vi "interfejsPC.vi"() -> ()   [LabVIEW 2014]
uses:
  glownaMaszynaStanowVIs/wczytajListePunktowVIs/RodzajPomiarow.ctl
  interfejsVIs/AkcjaInterfejsu.ctl
  glownaMaszynaStanowVIs/AkcjaGFV.ctl
  interfejsVIs/WejsciaVIs/WejsciaParametry.ctl
  interfejsVIs/WyjsciaVIs/WyjsciaParametry.ctl
panel:
  out "Połączono":bool
  in  "Połącz":bool
  in  "Port":u16=2000
  in  "Adres IP":string="192.168.0.102"
  in  "Wyjście":bool
  out "Odbiorcza azymut":i32
  out "Odbiorcza elewacja":i32
  out "Nadawcza azymut":i32
  out "Nadawcza elewacja":i32
  out "TCP Error":bool
  out "TCP Error Code":i32
  out "LINX Error Code":i32
  out "LINX Error":bool
  in  "Minimalna odległość":dbl=3.0
  in  "Długość ramienia":dbl=3.0
  in  "Testuj punkty":bool
  in  "Definicja punktów użytkownika:":i32[][](array[numeric])
  in  "Czas inicjalizacji ramion [s]":dbl=90.0
  in  "Czas pomiaru [s]":dbl=3.0
  in  "Rodzaj pomiarów:":T1
  out "Zrealizowano punkty:":string
  out "Pomiar":bool
  in  "Stop":bool
  in  "Start":bool
  out "Działanie ramienia":bool
  in  "Nadawcza/odbiorcza":bool
  out "Odb. góra":bool
  out "Odb. dół":bool
  out "Odb. prawo":bool
  out "Odb. lewo":bool
  in  "Dӣ":bool
  in  "GÓRA":bool
  in  "LEWO":bool
  in  "PRAWO":bool
  in  "Włącz/wyłącz":bool
  out "Nad. góra":bool
  out "Nad. dół":bool
  out "Nad. prawo":bool
  out "Nad. lewo":bool
  # "1. Podaj adres IP oraz port modułu sterującego. \nUstawione są domyślne wartości."
  # "Współrzędne kątowe ramion [st.]:"
  # "Informacje o błędach:"
  # "Ustawienia systemu.\nNajedź myszką na strzałki kontrolki aby\nprzeczytać opis."
  # "2. Wybierz rodzaj pomiarów:"
  # "3. Sprawdź ustawienia systemu i naciśnij \"Start\"."
  # "Komora nadawcza"
  # "Praca ręczna"
  # "Komora odbiorcza"
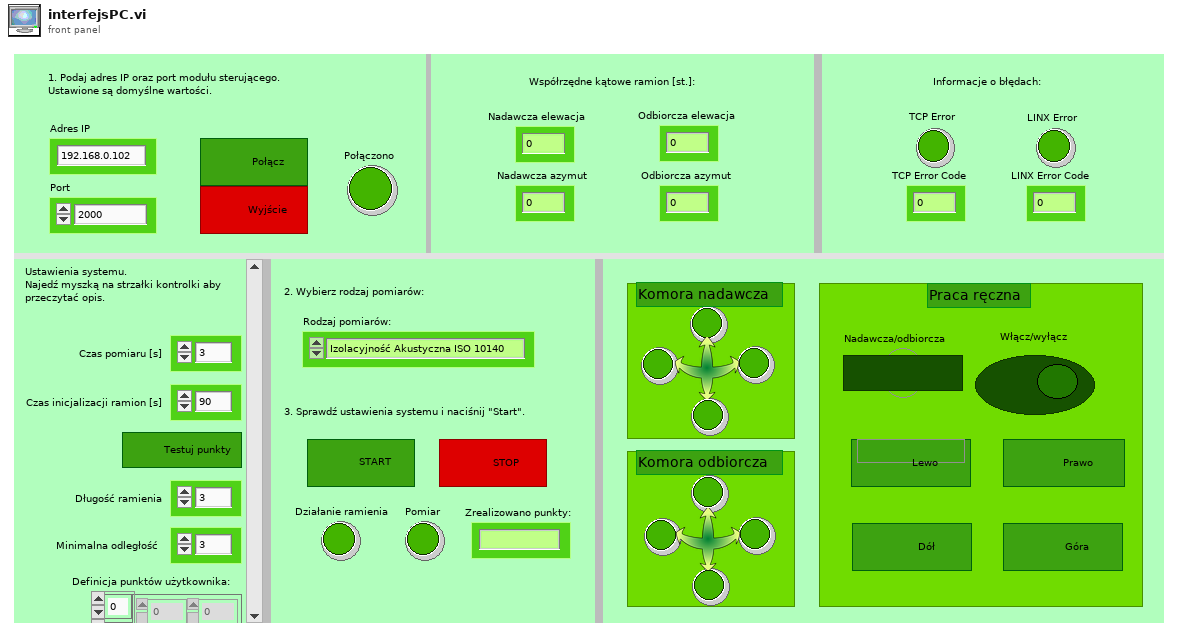
[diagram p1: front panel]
types:
  T1 = typedef "RodzajPomiarow.ctl" = enum16{"Izolacyjność Akustyczna ISO 10140", "Sekwencja testowa", "Definicja użytkownika"}
  T2 = typedef "AkcjaGFV.ctl" = enum16{"Czytaj", "Zapisz", "Reset"}
  T3 = typedef "AkcjaInterfejsu.ctl" = enum16{"Polacz", "Wczytaj", "Zapisz", "Koniec"}
  T4 = typedef "Odleglosc.ctl" = cluster{"Odległość [m]":dbl, "P1":i32[], "P2":i32[], "Czy poprawna":bool}
  T5 = typedef "WejsciaParametry.ctl" = cluster{"LEWO":bool, "PRAWO":bool, "GORA":bool, "DOL":bool, "Praca reczna":bool, "Stop":bool, "Start":bool, "Komora":bool, "Wyjscie":bool, "Rodzaj pomiarow":T1, "Czas pomiaru [s]":dbl, "Czas inicjalizacji ramion [s]":dbl, "Definicja punktów użytkownika":i32[][]}
  T6 = enum16{"Standard", "Buffered", "CRLF", "Immediate"}
  T7 = typedef "WyjsciaParametry.ctl" = cluster{"Nad. lewo":bool, "Nad.  prawo":bool, "Nad.  gora":bool, "Nad. doł":bool, "Dzialanie":bool, "Pomiar":bool, "Odb. lewo":bool, "Odb.  prawo":bool, "Odb.  gora":bool, "Odb. dol":bool, "Pozostalo punktow":i32, "Nad. elewacja":i32, "Nad. azymut":i32, "Odb. elewacja":i32, "Odb. azymut":i32, "TCP Error":bool, "TCP Error Code":i32, "LINX Error":bool, "LINX Error Code":i32}
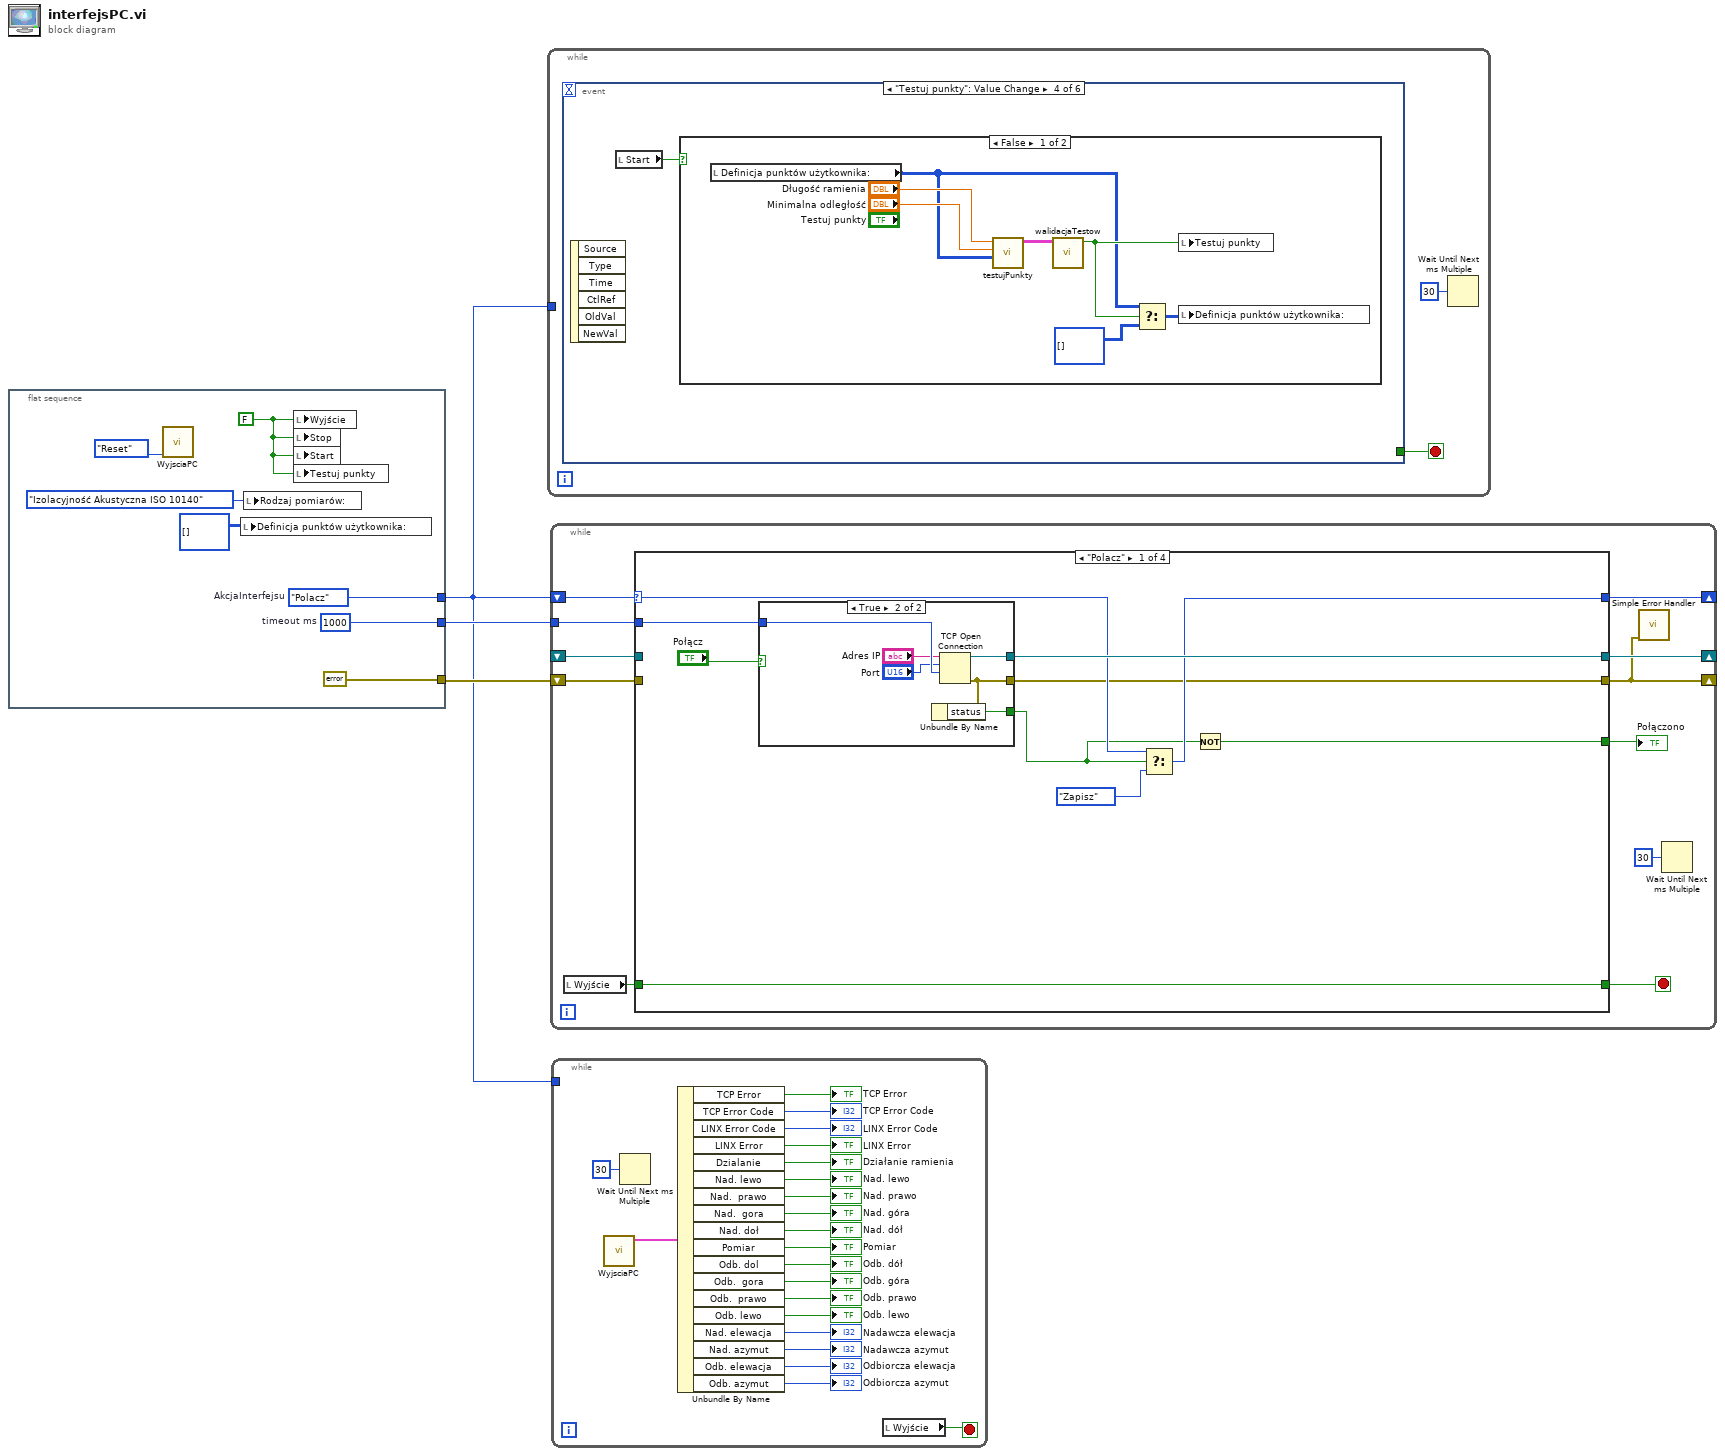
[diagram p0: block diagram]
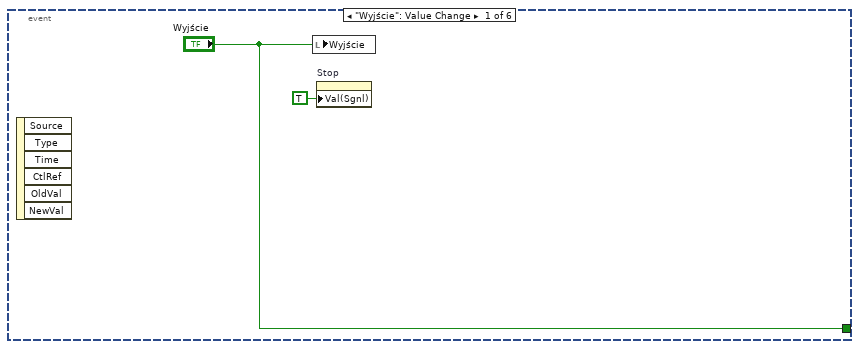
[diagram p2: hidden frame]
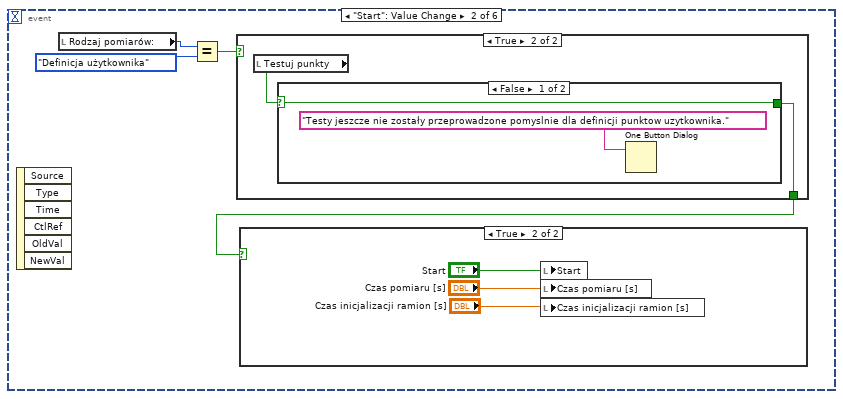
[diagram p3: hidden frame]
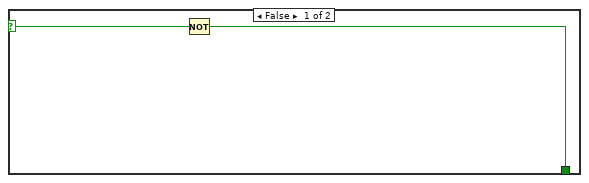
[diagram p5: hidden frame]
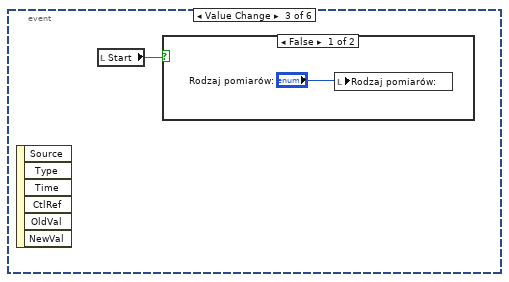
[diagram p7: hidden frame]
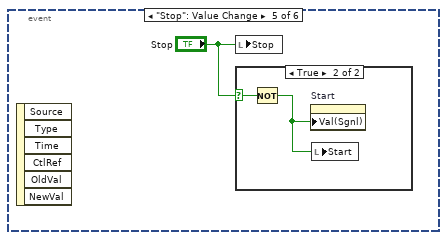
[diagram p10: hidden frame]
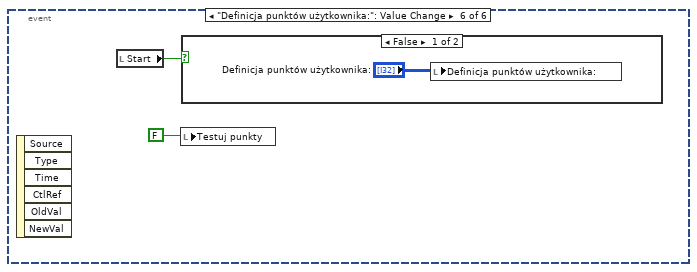
[diagram p12: hidden frame]
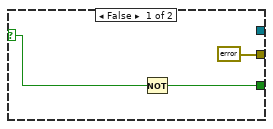
[diagram p14: hidden frame]
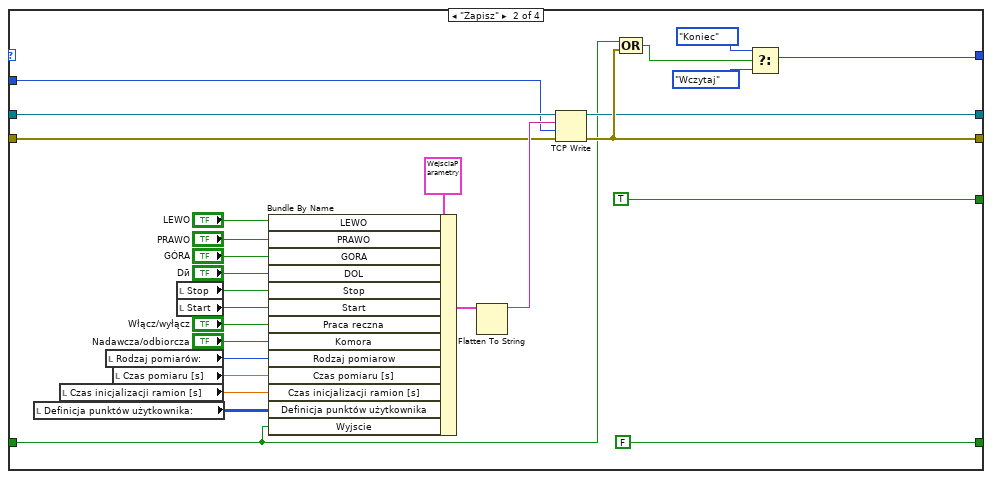
[diagram p15: hidden frame]
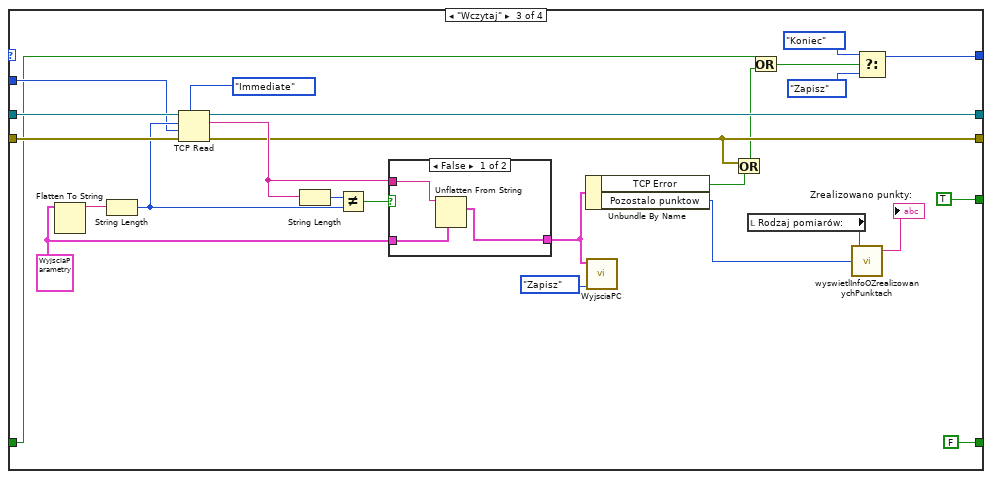
[diagram p16: hidden frame]
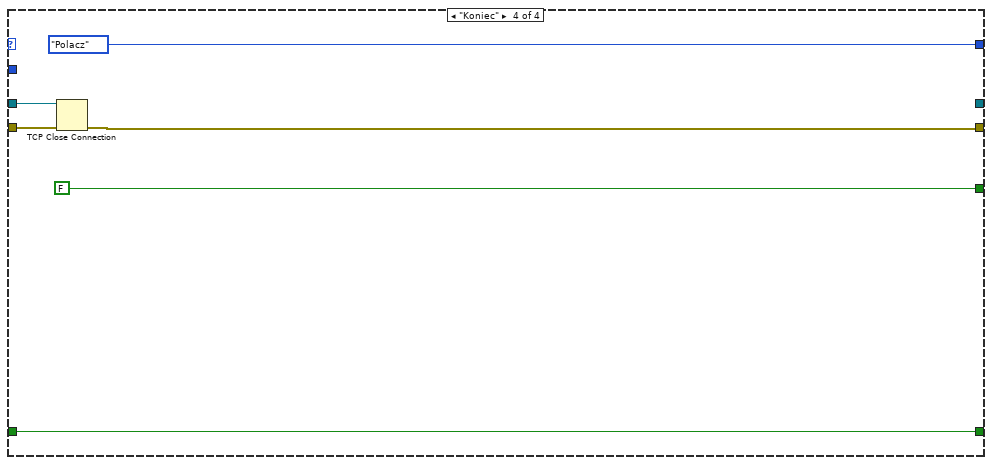
[diagram p18: hidden frame]
diagram:
  n1 = flat-sequence {
    tunnel: [w10] -> w1
    tunnel: [w9] -> w3
    tunnel: [errorcluster {"status"=FALSE, "code"=0, "source"=""} ("error out")] -> w2
    frame #0 {
      w5 = FALSE ("Wyjście")
      w9 = 1000  # timeout ms
      w10 = AkcjaInterfejsu."Polacz"  # AkcjaInterfejsu
      n2 = call "WyjsciaPC.vi"("Akcja"=AkcjaGFV."Reset") -> ()  [unwired: 10 in, 1 out]
      n3 = local write "Definicja punktów użytkownika:"(i32[][] [] ("Definicja punktów użytkownika")) -> ()
      n4 = local write "Rodzaj pomiarów:"(RodzajPomiarow."Izolacyjność Akustyczna ISO 10140" ("Rodzaj pomiarów:")) -> ()
      n5 = local write "Wyjście"(w5) -> ()
      n6 = local write "Stop"(w5) -> ()
      n7 = local write "Start"(w5) -> ()
      n8 = local write "Testuj punkty"(w5) -> ()
    }
  }
  n9 = while {
    tunnel: w1 -> [_]
    stop <- w12 stop-if-true
    n10 = event shown="[3] \"Testuj punkty\": Value Change" {
      selector: _ -> [_ _ _ _ _ _]
      dyn-events: _ -> [_ _ _ _ _ _]
      timeout: _ -> [_ _ _ _ _ _]
      tunnel: ["Wyjście" _ _ _ _ _] -> w12
      event "Wyjście": Value Change {
        n11 = event-data() -> ()  [unwired: 1 in, 6 out]
        n12 = local write "Wyjście"("Wyjście") -> ()
        n13 = property on="Stop" class="Bool (strict)"("Val(Sgnl)"=TRUE ("Value (Signaling)")) -> ()  [unwired: 2 in, 2 out]
      }
      event "Start": Value Change {
        n14 = event-data() -> ()  [unwired: 1 in, 6 out]
        n15 = local read "Rodzaj pomiarów:"() -> (w18:T1)
        n16 = Equal?(x=w18, y=RodzajPomiarow."Definicja użytkownika") -> (x = y?=w16:bool)
        n17 = case shown="True" w16 {
          selector: w16 -> [w23 _]
          tunnel: [w22 w24] -> w15
          frame False {
            n18 = Not(x=w23) -> (.not. x?=w22:bool)
          }
          frame True {
            n19 = local read "Testuj punkty"() -> (w25:bool)
            n20 = case shown="False" w25 {
              selector: w25 -> [w26 w28]
              tunnel: [w26 w28] -> w24
              frame False {
                n21 = One Button Dialog(message="Testy jeszcze nie zostały przeprowadzone pomyslnie dla definicji punktow uzytkownika.") -> ()  [unwired: 1 in, 1 out]
              }
              frame True {
              }
            }
          }
        }
        n22 = case shown="True" w15 {
          frame False {
          }
          frame True {
            n23 = local write "Start"("Start") -> ()
            n24 = local write "Czas pomiaru [s]"("Czas pomiaru [s]") -> ()
            n25 = local write "Czas inicjalizacji ramion [s]"("Czas inicjalizacji ramion [s]") -> ()
          }
        }
      }
      event Value Change {
        n26 = event-data() -> ()  [unwired: 1 in, 6 out]
        n27 = local read "Start"() -> (w29:bool)
        n28 = case shown="False" w29 {
          frame False {
            n29 = local write "Rodzaj pomiarów:"("Rodzaj pomiarów:") -> ()
          }
          frame True {
          }
        }
      }
      event "Testuj punkty": Value Change {
        n30 = event-data() -> ()  [unwired: 1 in, 6 out]
        n31 = local read "Start"() -> (w31:bool)
        n32 = case shown="False" w31 {
          frame False {
            n33 = local read "Definicja punktów użytkownika:"() -> (w32:i32[][])
            n34 = call "testujPunkty.vi"("Punkty"=w32, "Minimalna odległość"="Minimalna odległość", "Promień [m]"="Długość ramienia") -> ("Odleglosci"=w36:T4[][])  [unwired: 8 in]
            n35 = call "walidacjaTestow.vi"("Odleglosci"=w36) -> ("Testy przeszły?"=w35:bool)  [unwired: 10 in]
            n36 = Select(t=w32, s=w35, f=i32[][] []) -> (s? t:f=w33:i32[][])
            n37 = local write "Testuj punkty"(w35) -> ()
            n38 = local write "Definicja punktów użytkownika:"(w33) -> ()
          }
          frame True {
          }
        }
      }
      event "Stop": Value Change {
        n39 = event-data() -> ()  [unwired: 1 in, 6 out]
        n40 = local write "Stop"("Stop") -> ()
        n41 = case shown="True" "Stop" {
          selector: "Stop" -> [_ w41]
          frame False {
          }
          frame True {
            n42 = Not(x=w41) -> (.not. x?=w40:bool)
            n43 = property on="Start" class="Bool (strict)"("Val(Sgnl)"=w40) -> ()  [unwired: 2 in, 2 out]
            n44 = local write "Start"(w40) -> ()
          }
        }
      }
      event "Definicja punktów użytkownika:": Value Change {
        n45 = event-data() -> ()  [unwired: 1 in, 6 out]
        n46 = local read "Start"() -> (w42:bool)
        n47 = local write "Testuj punkty"(FALSE ("Testuj punkty")) -> ()
        n48 = case shown="False" w42 {
          frame False {
            n49 = local write "Definicja punktów użytkownika:"("Definicja punktów użytkownika:") -> ()
          }
          frame True {
          }
        }
      }
    }
    n50 = Wait Until Next ms Multiple(millisecond multiple=u32 30) -> ()  [unwired: 1 out]
  }
  n51 = while {
    shift-right: [w54] -> _
    shift-left: _ -> [w55]
    shift-right: [w46] -> _
    shift-left: w2 -> [w53]
    shift-right: [w49] -> _
    shift-left: w1 -> [w51]
    tunnel: w3 -> [w50]
    stop <- w52 stop-if-true
    n52 = local read "Wyjście"() -> (w48:bool)
    n53 = case shown="\"Polacz\"" w51 {
      selector: w51 -> [w60 _ _ _]
      tunnel: w55 -> [_ w101 w123 w137]
      tunnel: [w65 w85 w120 _] -> w54
      tunnel: [w57 w86 w109 w132] -> w46
      tunnel: w53 -> [_ w91 w124 w136]
      tunnel: [w63 FALSE ("Dzialanie") FALSE ("Wyjście") w134] -> w52
      tunnel: [w61 w90 w113 AkcjaInterfejsu."Polacz" ("AkcjaInterfejsu")] -> w49
      tunnel: w48 -> [w63 w75 w108 w134]
      tunnel: w50 -> [w62 w87 w121 _]
      tunnel: [w58 TRUE ("Wyjście") TRUE ("Wyjście") FALSE ("Wyjście")] -> w47
      frame "Polacz" {
        n54 = case shown="True" "Połącz" {
          selector: "Połącz" -> [w68 _]
          tunnel: [_ w74] -> w65
          tunnel: [errorcluster {"status"=FALSE, "code"=0, "source"=""} ("error out") w69] -> w57
          tunnel: w62 -> [_ w73]
          tunnel: [w66 w70] -> w56
          frame False {
            n55 = Not(x=w68) -> (.not. x?=w66:bool)
          }
          frame True {
            n56 = TCP Open Connection(address="Adres IP", remote port or service name="Port", timeout ms (60000)=w73) -> (connection ID=w74:refnum<k5>, error out=w69:errorcluster)  [unwired: 2 in]
            n57 = Unbundle By Name(w69) -> ("status"=w70:bool)
          }
        }
        n58 = Select(t=w60, s=w56, f=AkcjaInterfejsu."Zapisz" ("AkcjaInterfejsu")) -> (s? t:f=w61:T3)
        n59 = Not(x=w56) -> (.not. x?=w58:bool)
      }
      frame "Zapisz" {
        n60 = local read "Definicja punktów użytkownika:"() -> (w76:i32[][])
        n61 = local read "Czas inicjalizacji ramion [s]"() -> (w77:dbl)
        n62 = local read "Rodzaj pomiarów:"() -> (w82:T1)
        n63 = local read "Czas pomiaru [s]"() -> (w78:dbl)
        n64 = local read "Stop"() -> (w81:bool)
        n65 = local read "Start"() -> (w83:bool)
        n66 = Bundle By Name(cluster=T5 {"LEWO"=FALSE, "PRAWO"=FALSE, "GORA"=FALSE, "DOL"=FALSE, "Praca reczna"=FALSE, "Stop"=FALSE, "Start"=FALSE, "Komora"=FALSE, "Wyjscie"=FALSE, "Rodzaj pomiarow"=enum."Izolacyjność Akustyczna ISO 10140", "Czas pomiaru [s]"=2.0, "Czas inicjalizacji ramion [s]"=2.0, "Definicja punktów użytkownika"=[]} ("Wejścia interfejsu"), "LEWO"="LEWO", "PRAWO"="PRAWO", "GORA"="GÓRA", "DOL"="Dӣ", "Stop"=w81, "Start"=w83, "Praca reczna"="Włącz/wyłącz", "Komora"="Nadawcza/odbiorcza", "Rodzaj pomiarow"=w82, "Czas pomiaru [s]"=w78, "Czas inicjalizacji ramion [s]"=w77, "Definicja punktów użytkownika"=w76, "Wyjscie"=w75) -> (w93:T5)
        n67 = Flatten To String(anything=w93) -> (data string=w92:string)  [unwired: 3 in, 2 out]
        n68 = TCP Write(connection ID=w101, data in=w92, error in (no error)=w91, 9:w87) -> (connection ID out=w85:refnum<k5>, error out=w86:errorcluster)  [unwired: 1 out]
        n69 = Compound Arithmetic op=OR(w75, w86) -> (w88:bool)
        n70 = Select(t=AkcjaInterfejsu."Koniec", s=w88, f=AkcjaInterfejsu."Wczytaj") -> (s? t:f=w90:T3)
      }
      frame "Wczytaj" {
        w116 = T7 {"Nad. lewo"=FALSE, "Nad.  prawo"=FALSE, "Nad.  gora"=FALSE, "Nad. doł"=FALSE, "Dzialanie"=FALSE, "Pomiar"=FALSE, "Odb. lewo"=FALSE, "Odb.  prawo"=FALSE, "Odb.  gora"=FALSE, "Odb. dol"=FALSE, "Pozostalo punktow"=0, "Nad. elewacja"=0, "Nad. azymut"=0, "Odb. elewacja"=0, "Odb. azymut"=0, "TCP Error"=FALSE, "TCP Error Code"=0, "LINX Error"=FALSE, "LINX Error Code"=0} ("Cluster")
        n71 = Flatten To String(anything=w116) -> (data string=w126:string)  [unwired: 3 in, 2 out]
        n72 = String Length(string=w126) -> (length=w122:i32)
        n73 = TCP Read(connection ID=w123, bytes to read=w122, error in (no error)=w124, 7:T6."Immediate" ("mode (standard)"), 9:w121) -> (connection ID out=w120:refnum<k5>, data out=w117:string, error out=w109:errorcluster)
        n74 = String Length(string=w117) -> (length=w125:i32)
        n75 = Not Equal?(x=w125, y=w122) -> (x != y?=w118:bool)
        n76 = case shown="False" w118 {
          tunnel: w117 -> [w129 _]
          tunnel: w116 -> [w130 w131]
          tunnel: [w128 w131] -> w104
          frame False {
            n77 = Unflatten From String(type=w130, binary string=w129) -> (value=w128:T7)  [unwired: 3 in, 2 out]
          }
          frame True {
          }
        }
        n78 = Unbundle By Name(w104) -> ("TCP Error"=w103:bool, "Pozostalo punktow"=w102:i32)
        n79 = call "WyjsciaPC.vi"("Akcja"=AkcjaGFV."Zapisz", "Wejście"=w104) -> ()  [unwired: 9 in, 1 out]
        n80 = Or(x=w109, y=w103) -> (x .or. y?=w106:bool)
        n81 = local read "Rodzaj pomiarów:"() -> (w110:T1)
        n82 = Or(x=w108, y=w106) -> (x .or. y?=w107:bool)
        n83 = call "wyswietlInfoOZrealizowanychPunktach.vi"("Pozostalo punktow"=w102, "Rodzaj pomiarow"=w110) -> ("Zrealizowane punkty info"=→"Zrealizowano punkty:":string)  [unwired: 3 in]
        n84 = Select(t=AkcjaInterfejsu."Koniec", s=w107, f=AkcjaInterfejsu."Zapisz") -> (s? t:f=w113:T3)
      }
      frame "Koniec" {
        n85 = TCP Close Connection(connection ID=w137, error in (no error)=w136) -> (error out=w132:errorcluster)  [unwired: 1 in, 1 out]
      }
    }
    "Połączono" <- w47
    n86 = call <vilib>:"Simple Error Handler.vi"("error in (no error)"=w46) -> ()  [unwired: 4 in, 5 out]
    n87 = Wait Until Next ms Multiple(millisecond multiple=u32 30) -> ()  [unwired: 1 out]
  }
  n88 = while {
    tunnel: w1 -> [_]
    stop <- w139 stop-if-true
    n89 = call "WyjsciaPC.vi"() -> ("Wyjście"=w141:T7)  [unwired: 11 in]
    n90 = Wait Until Next ms Multiple(millisecond multiple=u32 30) -> ()  [unwired: 1 out]
    n91 = Unbundle By Name(w141) -> ("TCP Error"=→"TCP Error":bool, "TCP Error Code"=→"TCP Error Code":i32, "LINX Error Code"=→"LINX Error Code":i32, "LINX Error"=→"LINX Error":bool, "Dzialanie"=→"Działanie ramienia":bool, "Nad. lewo"=→"Nad. lewo":bool, "Nad.  prawo"=→"Nad. prawo":bool, "Nad.  gora"=→"Nad. góra":bool, "Nad. doł"=→"Nad. dół":bool, "Pomiar"=→"Pomiar":bool, "Odb. dol"=→"Odb. dół":bool, "Odb.  gora"=→"Odb. góra":bool, "Odb.  prawo"=→"Odb. prawo":bool, "Odb. lewo"=→"Odb. lewo":bool, "Nad. elewacja"=→"Nadawcza elewacja":i32, "Nad. azymut"=→"Nadawcza azymut":i32, "Odb. elewacja"=→"Odbiorcza elewacja":i32, "Odb. azymut"=→"Odbiorcza azymut":i32)
    n92 = local read "Wyjście"() -> (w139:bool)
  }
